vi "TDMSAdv writeOfTime.vi"(5 "channel name":string, 7 "group name (Untitled)":string, 8 "error in (no error)":errorcluster, 10 "dataArray":timestamp[](array[timestamp]), 11 "TDMSAdv in":refnum<class "TDMSAdv.lvclass">) -> (0 "error out":errorcluster, 3 "TDMSAdv out":refnum<class "TDMSAdv.lvclass">)   [LabVIEW 2018, in "TDMSAdv.lvclass"]
uses:
  TDMSAdv.lvclass
  TDMSAdv.lvclass/TDMSAdv.ctl
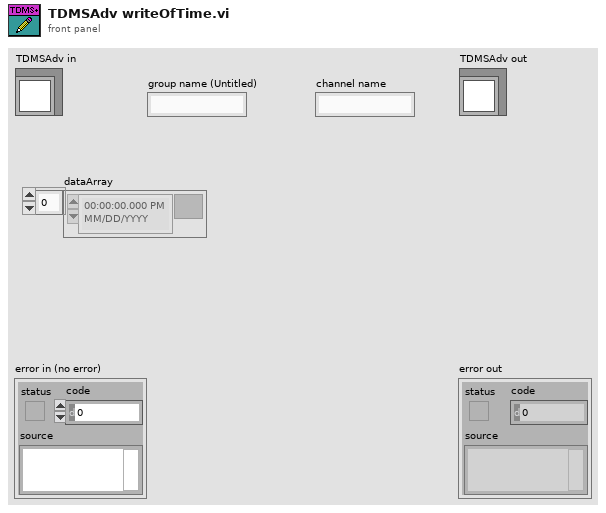
[diagram p1: front panel]
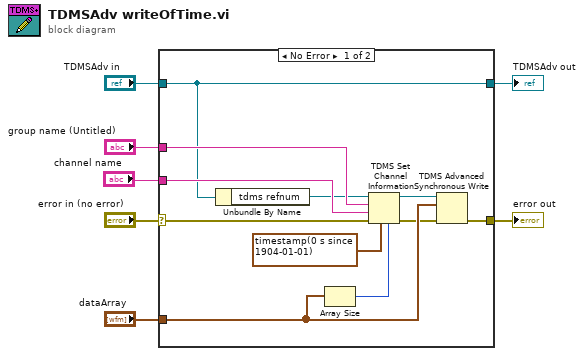
[diagram p0: block diagram]
diagram:
  n1 = case shown="No Error" "error in (no error)" {
    selector: "error in (no error)" -> [w16 w19]
    tunnel: "dataArray" -> [w17 _]
    tunnel: "group name (Untitled)" -> [w15 _]
    tunnel: "channel name" -> [w14 _]
    tunnel: "TDMSAdv in" -> [w12 w20]
    tunnel: [w12 w20] -> w3
    tunnel: [w11 w19] -> w2
    frame No Error {
      n2 = Unbundle By Name(w12) -> ("tdms refnum"=w13:refnum<k34>)
      n3 = Array Size(array=w17) -> (size(s)=w18:i32)
      n4 = TDMS Set Channel Information(4:w18, 6:timestamp(0 s since 1904-01-01), 8:w16, 9:w14, 10:w15, 11:w13) -> (0:w9:errorcluster, 3:w10:refnum<k34>)  [unwired: 1 in]
      n5 = TDMS Advanced Synchronous Write(8:w9, 10:w17, 11:w10) -> (0:w11:errorcluster)  [unwired: 1 out]
    }
    frame Error {
    }
  }
  "TDMSAdv out" <- w3
  "error out" <- w2
